vi "StartListener.vi"(0 "reference":refnum<class "VdTcpIP.lvclass">, 5 "error in (no error)":errorcluster, 7 "Debug(False)":bool) -> (14 "reference out":refnum<class "VdTcpIP.lvclass">, 19 "error out":errorcluster)   [LabVIEW 2020, in "VdTcpIP.lvclass"]
doc: "Starts a listener process, which waits for connections"
uses:
  VdTcpIP.lvclass
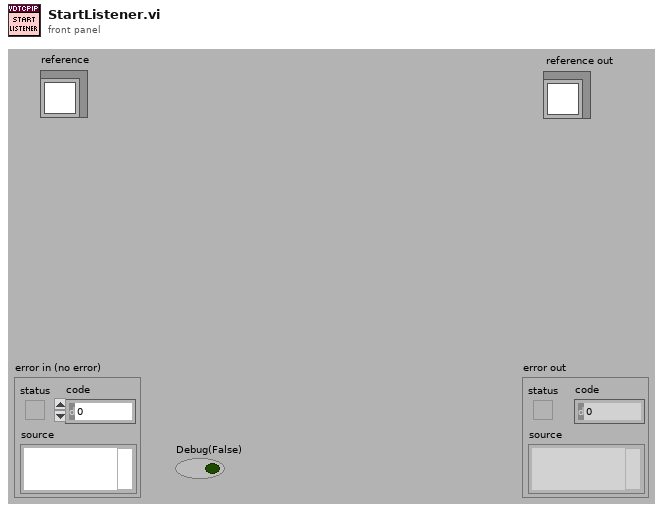
[diagram p1: front panel]
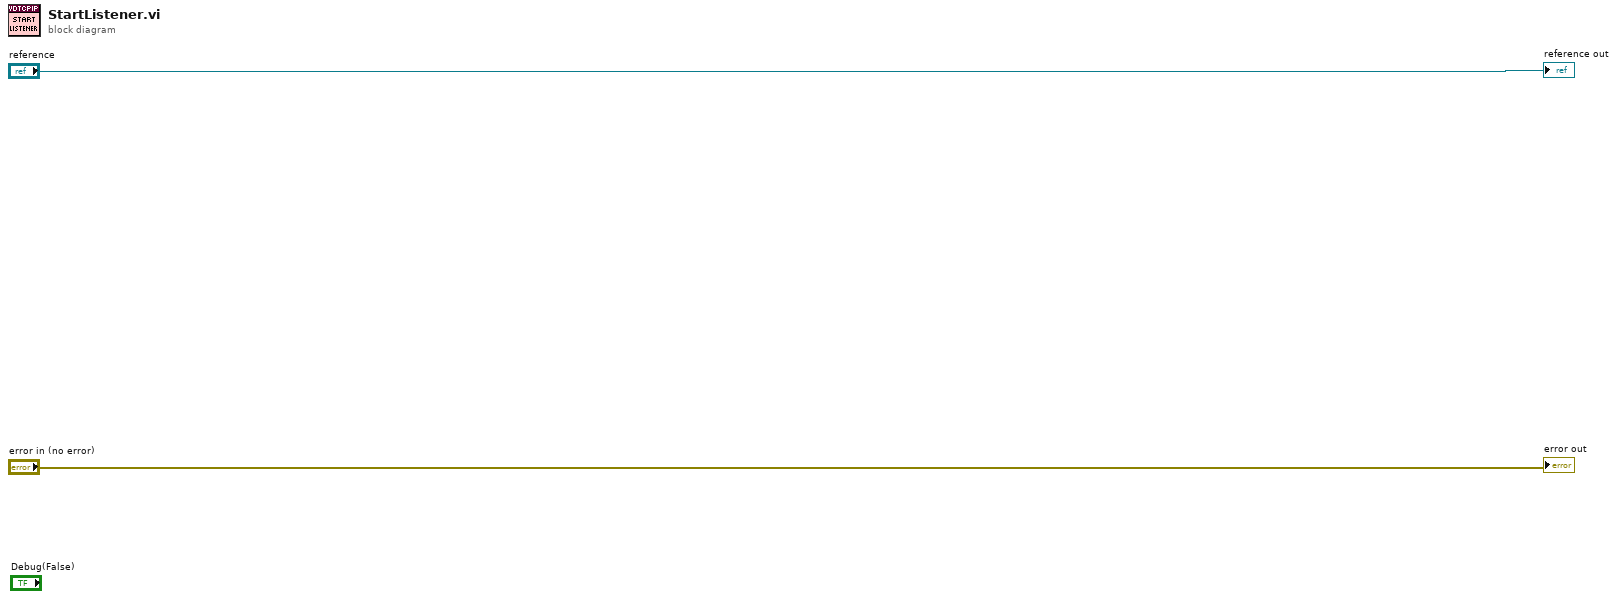
[diagram p0: block diagram]
diagram:
  "reference out" <- "reference"
  "error out" <- "error in (no error)"
